vi "Error Code.vi"(8 "Error in":errorcluster, 11 "Error code":i32) -> (0 "Error out":errorcluster)   [LabVIEW 2014, in "HDF5Tools.lvlib"]
uses:
  HDF5Tools.lvlib
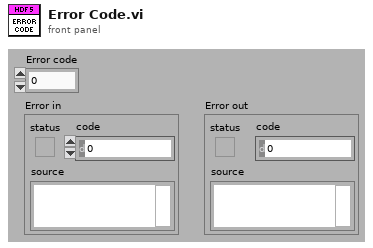
[diagram p1: front panel]
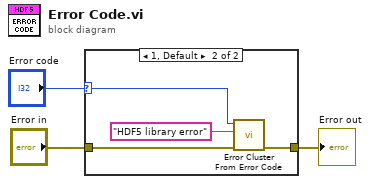
[diagram p0: block diagram]
diagram:
  n1 = case shown="1, Default" "Error code" {
    selector: "Error code" -> [_ w7]
    tunnel: "Error in" -> [w4 w6]
    tunnel: [w4 w5] -> w1
    frame 0 {
    }
    frame 1, Default {
      n2 = call <vilib>:"Error Cluster From Error Code.vi"("error in (no error)"=w6, "error message (\"\")"="HDF5 library error" ("error message (\"\")"), "error code (0)"=w7) -> ("error out"=w5:errorcluster)  [unwired: 6 in]
    }
  }
  "Error out" <- w1
